vi "read.vi"(6 "call chain index (1)":i32=1, 7 "vi ref (caller)":refnum<vi>, 8 "error in (no error)":errorcluster) -> (0 "error out":errorcluster, 1 "body":string[](array[string]), 2 "header":string[](array[string]), 3 "summary control id":i32, 4 "footer":string[](array[string]), 5 "summary text":string)   [LabVIEW 2024, in "summary manager.lvlib"]
uses:
  summary manager.lvlib
  <vilib>/Utility/error.llb/whitespace.ctl
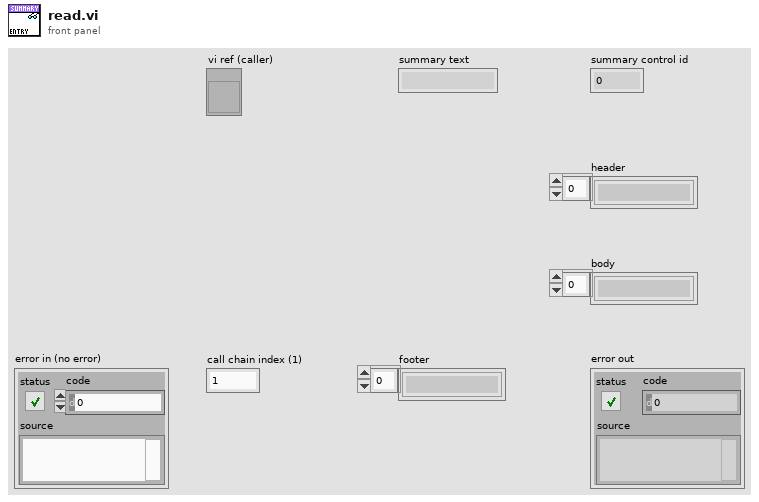
[diagram p1: front panel]
types:
  T1 = typedef "whitespace.ctl" = u16
  T2 = typedef "summary manager.lvlib/entry type.ctl" = cluster{"summary control id":i32, "header":string[], "body":string[], "footer":string[]}
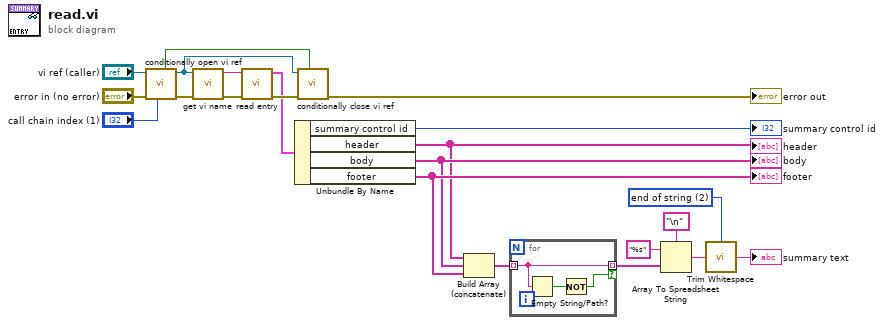
[diagram p0: block diagram]
diagram:
  w1 = T1 2 items=["both", "start of string", "end of string"]
  n1 = call "conditionally open vi ref.vi"("call chain index (1)"="call chain index (1)", "error in (no error)"="error in (no error)", "vi ref in"="vi ref (caller)") -> ("error out"=w21:errorcluster, "vi ref out"=w18:refnum<vi>, "new ref?"=w17:bool)  [unwired: 6 in]
  n2 = call "get vi name.vi"("error in (no error)"=w21, "vi ref"=w18) -> ("error out"=w14:errorcluster, "vi name"=w12:string)  [unwired: 8 in]
  n3 = call "read entry.vi"("error in (no error)"=w14, "id"=w12) -> ("error out"=w13:errorcluster, "entry"=w11:T2)  [unwired: 8 in]
  n4 = Unbundle By Name(w11) -> ("summary control id"=→"summary control id":i32, "header"=w5:string[], "body"=w9:string[], "footer"=w22:string[])
  "header" <- w5
  "body" <- w9
  "footer" <- w22
  n5 = call "conditionally close vi ref.vi"("new ref?"=w17, "error in (no error)"=w13, "vi ref"=w18) -> ("error out"=→"error out":errorcluster)  [unwired: 8 in]
  n6 = Build Array (concatenate)(w5, w9, w22) -> (w4:string[])
  n7 = for {
    tunnel: w4 -> [w25] mode=indexing
    tunnel: [w25] -> w3 mode=indexing if=w23
    n8 = Empty String/Path?(string/path=w25) -> (empty?=w24:bool)
    n9 = Not(x=w24) -> (.not. x?=w23:bool)
  }
  n10 = Array To Spreadsheet String(delimiter (Tab)="\n", array=w3, 3:"%s") -> (spreadsheet string=w6:string)
  n11 = call <vilib>:"Trim Whitespace.vi"("string"=w6, "location (both)"=w1) -> ("trimmed string"=→"summary text":string)
